vi "Triangle Waveform.vi"(5 "offset":dbl format="%0.2p", 6 "sampling info":cluster{"Fs":dbl, "#s":dbl}={"Fs"=1000.0, "#s"=1000.0} {"Fs" format="%.2p"}, 7 "reset signal":bool, 8 "error in (no error)":errorcluster, 9 "phase":dbl format="%.2p", 10 "amplitude":dbl=1.0 format="%0.2p", 11 "frequency":dbl=10.0 format="%0.2p") -> (0 "error out":errorcluster, 3 "signal out":waveform(dbl))   [LabVIEW 2009]
doc: "Generates a waveform containing a triangle wave."
uses:
  ma_Updatet0 timestamp.vi
  <vilib>/measure/NI_MABase.lvlib
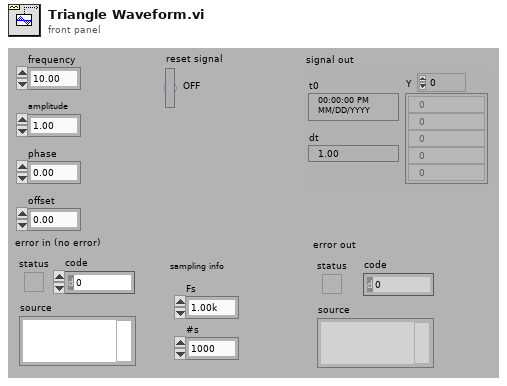
[diagram p1: front panel]
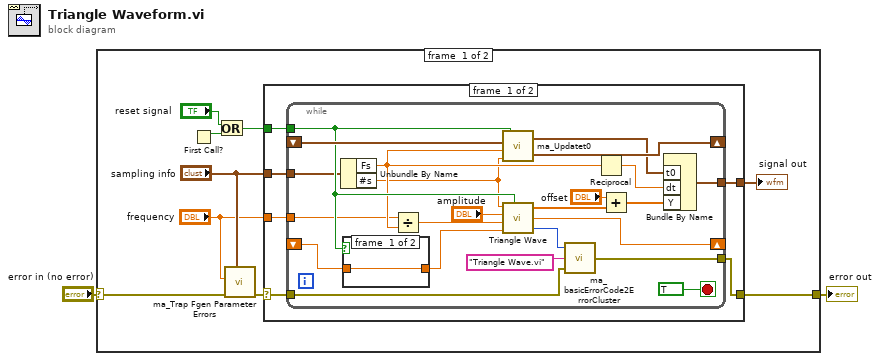
[diagram p0: block diagram]
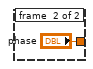
[diagram p2: hidden frame]
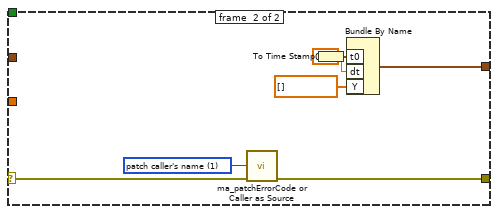
[diagram p3: hidden frame]
diagram:
  n1 = case shown="No Error" "error in (no error)" {
    selector: "error in (no error)" -> [w3 w50]
    tunnel: [w5 w50] -> w2
    frame #0 {
      n2 = First Call?() -> (First Call?: T/F=w9:bool)
      n3 = Or(x="reset signal", y=w9) -> (x .or. y?=w10:bool)
      n4 = call "ma_Trap Fgen Parameter Errors.vi"("Sampling info"="sampling info", "error in (no error)"=w3, "frequency"="frequency") -> ("error out"=w8:errorcluster)  [unwired: 8 in]
      n5 = case shown="No Error" w8 {
        selector: w8 -> [w12 w45]
        tunnel: w10 -> [w17 _]
        tunnel: "sampling info" -> [w16 _]
        tunnel: "frequency" -> [w15 _]
        tunnel: [w14 w43] -> w5
        tunnel: [w13 w47] -> w4
        frame #0 {
          n6 = while {
            tunnel: w12 -> [w19]
            tunnel: [w20] -> w13
            tunnel: [w21] -> w14
            tunnel: w15 -> [w22]
            tunnel: w16 -> [w23]
            tunnel: w17 -> [w27]
            shift-left: _ -> [w30]
            shift-right: [w32] -> _
            shift-left: _ -> [w37]
            shift-right: [w36] -> _
            stop <- TRUE stop-if-true
            n7 = Unbundle By Name(w23) -> ("Fs"=w25:dbl, "#s"=w24:dbl)
            n8 = case shown="True" w27 {
              tunnel: [w41 "phase"] -> w31
              tunnel: w30 -> [w41 _]
              frame #0 {
              }
              frame #1 {
              }
            }
            n9 = Divide(x=w22, y=w25) -> (x/y=w26:dbl)
            n10 = call-poly "ma_Updatet0.vi"("samples"=w24, "sampling rate (S/s)"=w25, "tf previous"=w37, "Reset Generation"=w27) -> ("tf new"=w36:timestamp, "t0"=w18:timestamp)
            n11 = call "Triangle Wave.vi"("samples"=w24, "amplitude"="amplitude", "f"=w26, "phase in"=w31, "reset phase"=w27) -> ("triangle wave"=w34:dbl[], "phase out"=w32:dbl, "error"=w40:i32)
            n12 = call <vilib>:"ma_basicErrorCode2ErrorCluster.vi"("error in (no error)"=w19, "subVI name"="Triangle Wave.vi" ("subVI Name"), "Error Code"=w40) -> ("error out"=w21:errorcluster)
            n13 = Reciprocal(x=w25) -> (1/x=w29:dbl)
            n14 = Add(x="offset", y=w34) -> (x+y=w33:dbl[])
            n15 = Bundle By Name("t0"=w18, "dt"=w29, "Y"=w33) -> (w20:waveform(dbl))  [unwired: 1 in]
          }
        }
        frame #1 {
          w44 = u16 1 items=["patch error code", "patch caller's name"] ("operation")
          w49 = 0.0 ("t0")
          n16 = call "ma_patchErrorCode or Caller as Source.vi"("error in (no error)"=w45, "operation"=w44) -> ("error out"=w43:errorcluster)  [unwired: 9 in]
          n17 = To Time Stamp(1:w49) -> (0:w46:timestamp)
          n18 = Bundle By Name("t0"=w46, "dt"=w49, "Y"=dbl[] []) -> (w47:waveform(dbl))  [unwired: 1 in]
        }
      }
      "signal out" <- w4
    }
    frame #1 {
    }
  }
  "error out" <- w2
